vi "Create Convenience Kernel.vi"(7 "Kernel Name":string, 8 "error in (no error)":errorcluster, 9 "Program Handle":T1, 10 "Preferred Vector Size 32f":u32, 11 "Device ID":T2) -> (0 "error out":errorcluster, 1 "Kernel Handle":T3)   [LabVIEW 2012]
uses:
  Controls/Kernel Handle.ctl
  Controls/Device ID.ctl
  Controls/Program Handle.ctl
  OpenCLV x64.lvlib
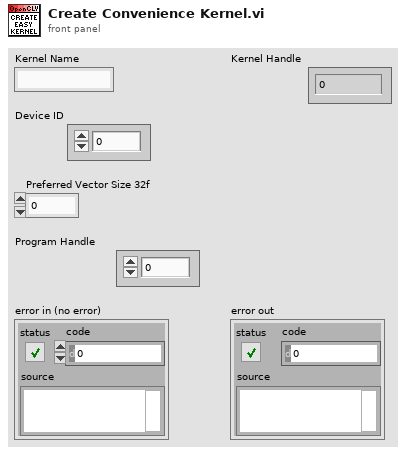
[diagram p1: front panel]
types:
  T1 = typedef "OpenCLV x64.lvlib/Program Handle.ctl" = u64
  T2 = typedef "OpenCLV x64.lvlib/Device ID.ctl" = u64
  T3 = typedef "OpenCLV x64.lvlib/Kernel Handle.ctl" = u64
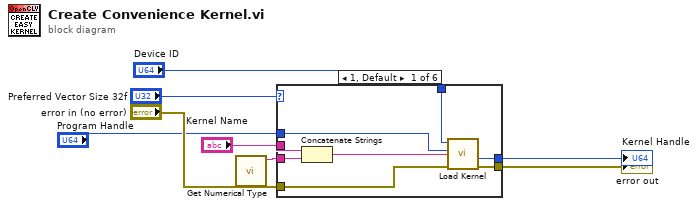
[diagram p0: block diagram]
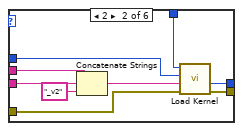
[diagram p2: hidden frame]
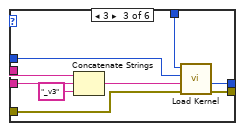
[diagram p3: hidden frame]
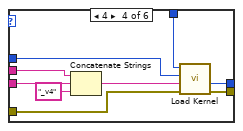
[diagram p4: hidden frame]
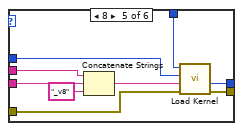
[diagram p5: hidden frame]
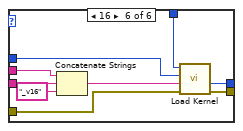
[diagram p6: hidden frame]
diagram:
  n1 = call "Get Numerical Type.vi"() -> ("VI Numerical Type"=w7:string)  [unwired: 11 in]
  n2 = case shown="1, Default" "Preferred Vector Size 32f" {
    tunnel: [w16 w25 w34 w43 w52 w61] -> w1
    tunnel: "Program Handle" -> [w15 w24 w33 w42 w51 w60]
    tunnel: w7 -> [w14 w22 w31 w39 w49 w57]
    tunnel: "Kernel Name" -> [w13 w23 w30 w40 w48 w58]
    tunnel: "error in (no error)" -> [w10 w18 w27 w36 w45 w54]
    tunnel: "Device ID" -> [w11 w19 w28 w37 w46 w55]
    tunnel: [w9 w17 w26 w35 w44 w53] -> w8
    frame 1, Default {
      n3 = Concatenate Strings(w13, w14) -> (w12:string)
      n4 = call "Load Kernel.vi"("Error In"=w10, "Kernel Name"=w12, "Program Handle"=w15, "Device In"=w11) -> ("Error Out"=w16:errorcluster, "Kernel Handle"=w9:T3)  [unwired: 4 in, 2 out]
    }
    frame 2 {
      n5 = Concatenate Strings(w23, w22, "_v2" ("string")) -> (w20:string)
      n6 = call "Load Kernel.vi"("Error In"=w18, "Kernel Name"=w20, "Program Handle"=w24, "Device In"=w19) -> ("Error Out"=w25:errorcluster, "Kernel Handle"=w17:T3)  [unwired: 4 in, 2 out]
    }
    frame 3 {
      n7 = Concatenate Strings(w30, w31, "_v3" ("string")) -> (w29:string)
      n8 = call "Load Kernel.vi"("Error In"=w27, "Kernel Name"=w29, "Program Handle"=w33, "Device In"=w28) -> ("Error Out"=w34:errorcluster, "Kernel Handle"=w26:T3)  [unwired: 4 in, 2 out]
    }
    frame 4 {
      n9 = Concatenate Strings(w40, w39, "_v4" ("string")) -> (w38:string)
      n10 = call "Load Kernel.vi"("Error In"=w36, "Kernel Name"=w38, "Program Handle"=w42, "Device In"=w37) -> ("Error Out"=w43:errorcluster, "Kernel Handle"=w35:T3)  [unwired: 4 in, 2 out]
    }
    frame 8 {
      n11 = Concatenate Strings(w48, w49, "_v8" ("string")) -> (w47:string)
      n12 = call "Load Kernel.vi"("Error In"=w45, "Kernel Name"=w47, "Program Handle"=w51, "Device In"=w46) -> ("Error Out"=w52:errorcluster, "Kernel Handle"=w44:T3)  [unwired: 4 in, 2 out]
    }
    frame 16 {
      n13 = Concatenate Strings(w58, w57, "_v16" ("string")) -> (w56:string)
      n14 = call "Load Kernel.vi"("Error In"=w54, "Kernel Name"=w56, "Program Handle"=w60, "Device In"=w55) -> ("Error Out"=w61:errorcluster, "Kernel Handle"=w53:T3)  [unwired: 4 in, 2 out]
    }
  }
  "Kernel Handle" <- w8
  "error out" <- w1
